vi "Send Command.vi"(8 "error in (no error)":errorcluster, 9 "Expected Response":string, 10 "Command":string, 11 "Simulated Serial Device":refnum<class "Simulated Serial Device.lvclass">) -> (0 "error out":errorcluster, 2 "read buffer":string, 3 "Simulated Serial Device Out":refnum<class "Simulated Serial Device.lvclass">)   [LabVIEW 2017, in "Simulated Serial Device.lvclass"]
uses:
  Simulated Serial Device.lvclass
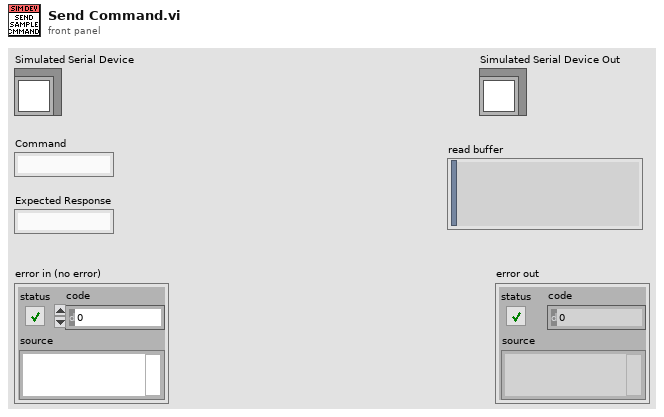
[diagram p1: front panel]
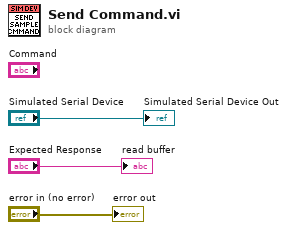
[diagram p0: block diagram]
diagram:
  "error out" <- "error in (no error)"
  "Simulated Serial Device Out" <- "Simulated Serial Device"
  "read buffer" <- "Expected Response"
